vi "buildtest.vi"   [LabVIEW 2019]
uses:
  PostBuildSupport/PostBuildSupport.lvclass
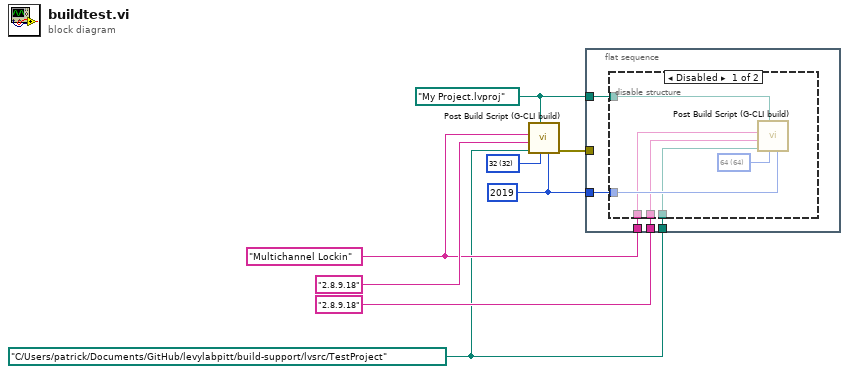
[diagram p0: block diagram]
diagram:
  w1 = path "C:/Users/patrick/Documents/GitHub/levylabpitt/build-support/lvsrc/TestProject" ("Package Source Folder")
  w2 = "Multichannel Lockin" ("Product Name")
  w6 = u32 2019 ("LV Version")
  w8 = u32 32 items=["32"=32, "64"=64] ("Architecture")
  w7 = path "My Project.lvproj" ("Project File Path")
  n1 = call "Post Build Script (G-CLI build).vi"("LV Version"=w6, "Architecture"=w8, "Project File Path"=w7, "Package Source Folder"=w1, "Package Version"="2.8.9.18", "Product Name"=w2) -> ("error out"=w5:errorcluster)  [unwired: 5 in]
  n2 = flat-sequence {
    tunnel: w7 -> [w13]
    tunnel: w6 -> [w12]
    tunnel: w5 -> [_]
    tunnel: "2.8.9.18" ("Package Version") -> [w11]
    tunnel: w2 -> [w10]
    tunnel: w1 -> [w9]
    frame #0 {
      n3 = disable-structure shown="Disabled" {
        disable-tunnel: w13 -> [w19 _]
        disable-tunnel: w12 -> [w18 _]
        disable-tunnel: w11 -> [w16 _]
        disable-tunnel: w10 -> [w15 _]
        disable-tunnel: w9 -> [w14 _]
        frame Disabled {
          w17 = u32 64 items=["32"=32, "64"=64] ("Architecture")
          n4 = call "Post Build Script (G-CLI build).vi"("LV Version"=w18, "Architecture"=w17, "Project File Path"=w19, "Package Source Folder"=w14, "Package Version"=w16, "Product Name"=w15) -> ()  [unwired: 5 in, 1 out]
        }
        frame Enabled {
        }
      }
    }
  }
